vi "Receive Joystick Update.vi"(8 "error in (no error)":errorcluster, 10 "Joystick State":T1, 11 "Test-XBox Controller-Receive Updates in":refnum<class "Test-XBox Controller-Receive Updates.lvclass">) -> (0 "Joystick.lvlib:Joystick.lvclass:Joystick State.ctlerror out":errorcluster, 3 "Test-XBox Controller-Receive Updates out":refnum<class "Test-XBox Controller-Receive Updates.lvclass">)   [LabVIEW 2014, in "Comp XBox One Controller.lvlib" / "Test-XBox Controller-Receive Updates.lvclass"]
uses:
  Test-XBox Controller-Receive Updates.lvclass
  Robot/Joystick/Joystick Class/Joystick State.ctl
  Robot/Joystick/Joystick Class/Button State.ctl
  Robot/Joystick/Joystick Class/Axis State.ctl
  Test-XBox Controller-Receive Updates.lvclass/Test-XBox Controller-Receive Updates.ctl
  Robot/Joystick/Joystick Class/Joystick.lvclass
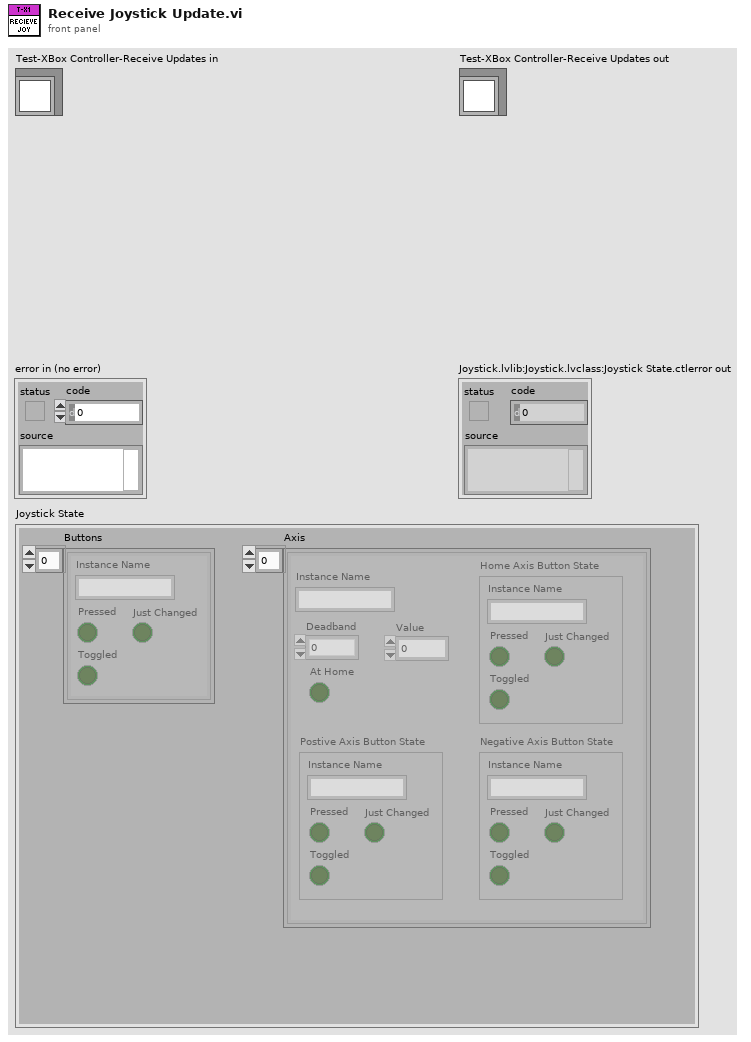
[diagram p1: front panel]
types:
  T1 = typedef "Joystick.lvlib/Joystick.lvclass/Joystick State.ctl" = cluster{"Buttons":T2[], "Axis":T3[]}
  T2 = typedef "Joystick.lvlib/Joystick.lvclass/Button State.ctl" = cluster{"Pressed":bool, "Instance Name":string, "Toggled":bool, "Just Changed":bool}
  T3 = typedef "Joystick.lvlib/Joystick.lvclass/Axis State.ctl" = cluster{"Instance Name":string, "Deadband":dbl, "Value":dbl, "At Home":bool, "Postive Axis Button State":T2, "Negative Axis Button State":T2, "Home Axis Button State":T2}
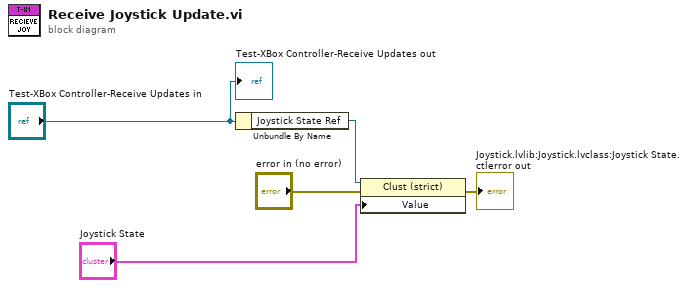
[diagram p0: block diagram]
diagram:
  n1 = Unbundle By Name("Test-XBox Controller-Receive Updates in") -> ("Joystick State Ref"=w4:refnum<vi>)
  n2 = property class="Clust (strict)"(reference=w4, error in="error in (no error)", "Value"="Joystick State") -> (error out=→"Joystick.lvlib:Joystick.lvclass:Joystick State.ctlerror out":errorcluster)  [unwired: 1 out]
  "Test-XBox Controller-Receive Updates out" <- "Test-XBox Controller-Receive Updates in"
